vi "FdxGetServerResourcesCvi.vi"(8 "error in":errorcluster, 11 "ServerRElement":u32) -> (0 "error out":errorcluster, 1 "ServerResourceInfo":T1 {"ResourceType" items=["RESOURCETYPE_BOARD"=0, "RESOURCETYPE_PORT"=1, "RESOURCETYPE_ALL"=20]}, 2 "ResourceType":u32(ring) items=["RESOURCETYPE_BOARD"=0, "RESOURCETYPE_PORT"=1, "RESOURCETYPE_ALL"=20], 3 "Resource ID":u32, 4 "StructId":u32, 5 "Resource Info":string)   [LabVIEW 2020, in "AIM664LV.lvlib"]
doc: "To get information from the server list about a resource."
uses:
  AIM664LV.lvlib
  FdxGlobalDllPath.vi
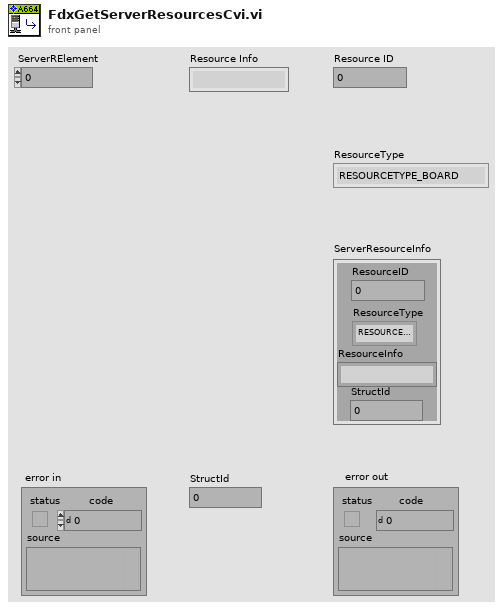
[diagram p1: front panel]
types:
  T1 = cluster{"ResourceID":u32, "ResourceType":u32, "ResourceInfo":string, "StructId":u32}
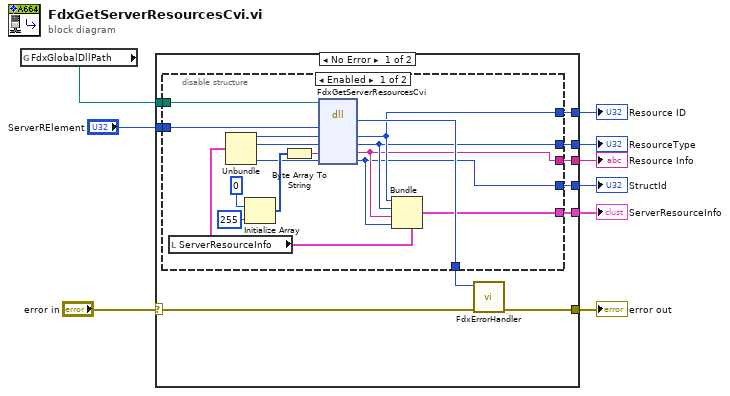
[diagram p0: block diagram]
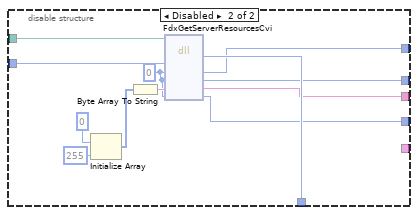
[diagram p2: hidden frame]
diagram:
  n1 = global read "FdxGlobalDllPath.vi" "FdxGlobalDllPath"() -> (w7:path)
  n2 = case shown="No Error" "error in" {
    selector: "error in" -> [w18 w48]
    tunnel: [w19 w48] -> w9
    tunnel: w7 -> [w16 _]
    tunnel: "ServerRElement" -> [w15 _]
    tunnel: [w14 _] -> w5
    tunnel: [w13 _] -> w4
    tunnel: [w12 _] -> w3
    tunnel: [w11 _] -> w2
    tunnel: [w10 _] -> w1
    frame No Error {
      n3 = disable-structure shown="Enabled" {
        disable-tunnel: [w35 w47] -> w17
        disable-tunnel: w16 -> [w26 w42]
        disable-tunnel: w15 -> [w25 w41]
        disable-tunnel: [w24 w40] -> w14
        disable-tunnel: [w23 w38] -> w13
        disable-tunnel: [w22 w37] -> w12
        disable-tunnel: [w21 w36] -> w11
        disable-tunnel: [w20 _] -> w10
        frame Enabled {
          n4 = local read "ServerResourceInfo"() -> (w27:T1)
          n5 = Unbundle(w27) -> ("ResourceID"=w30:u32, "ResourceType"=w29:u32, "StructId"=w28:u32)  [unwired: 1 out]
          n6 = Initialize Array(u8 0 ("ServerRElement"), 255 ("dimension size")) -> (w31:u8[])
          n7 = Byte Array To String(unsigned byte array=w31) -> (string=w32:string)
          n8 = dll-call lib="aim_fdx.19.dll" fn="FdxGetServerResourcesCvi"(path in=w26, "ServerRElement"=w25, "ResourceID"=w30, "ResourceType"=w29, "ResourceInfo"=w32, "StructId"=w28) -> ("status"=w35:i32, "ResourceID"=w24:u32, "ResourceType"=w23:u32, "ResourceInfo"=w22:string, "StructId"=w21:u32)  [unwired: 3 in, 2 out]
          n9 = Bundle(cluster=w27, "ResourceID"=w24, "ResourceType"=w23, "ResourceInfo"=w22, "StructId"=w21) -> (w20:T1)
        }
        frame Disabled {
          w39 = u32 0 ("ResourceID")
          n10 = Initialize Array(u8 0 ("ServerRElement"), 255 ("dimension size")) -> (w43:u8[])
          n11 = Byte Array To String(unsigned byte array=w43) -> (string=w44:string)
          n12 = dll-call lib="aim_fdx.19.dll" fn="FdxGetServerResourcesCvi"(path in=w42, "ServerRElement"=w41, "ResourceID"=w39, "ResourceType"=w39, "ResourceInfo"=w44, "StructId"=w39) -> ("status"=w47:i32, "ResourceID"=w40:u32, "ResourceType"=w38:u32, "ResourceInfo"=w37:string, "StructId"=w36:u32)  [unwired: 3 in, 2 out]
        }
      }
      n13 = call "FdxErrorHandler.vi"("error in"=w18, "AIM Error"=w17) -> ("error out"=w19:errorcluster)  [unwired: 9 in]
    }
    frame Error {
    }
  }
  "error out" <- w9
  "Resource Info" <- w3
  "Resource ID" <- w5
  "ResourceType" <- w4
  "StructId" <- w2
  "ServerResourceInfo" <- w1
